vi "Read Components.vi"(8 "error in (no error)":errorcluster, 11 "Snake in":refnum<class "Snake.lvclass">) -> (0 "error out":errorcluster, 2 "Components":T1[](array[typedef]), 3 "Snake out":refnum<class "Snake.lvclass">)   [LabVIEW 2019, in "Snake.lvclass"]
uses:
  Snake.lvclass
  Direction STYP.ctl
  Coordinate STYP.ctl
  private/Snake Component STYP.ctl
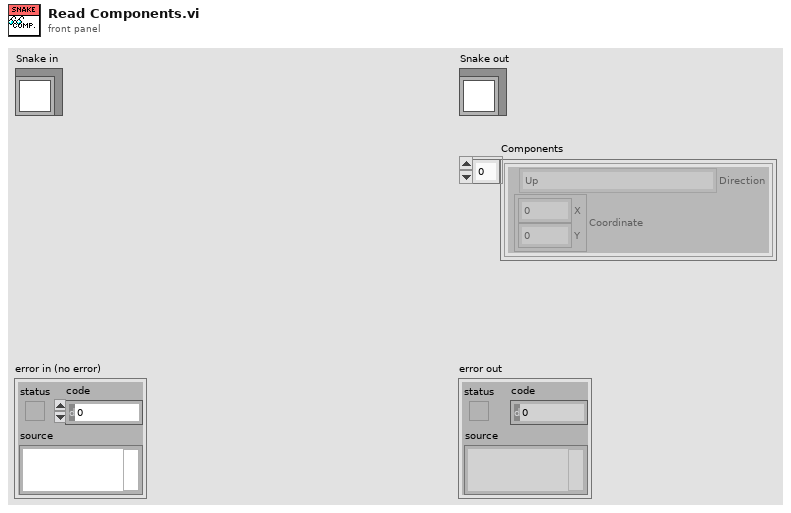
[diagram p1: front panel]
types:
  T1 = typedef "Snake.lvclass/Snake Component STYP.ctl" = cluster{"Direction":T2, "Coordinate":T3}
  T2 = typedef "Direction STYP.ctl" = enum16{"Up", "Down", "Left", "Right"}
  T3 = typedef "Coordinate STYP.ctl" = cluster{"X":i32, "Y":i32}
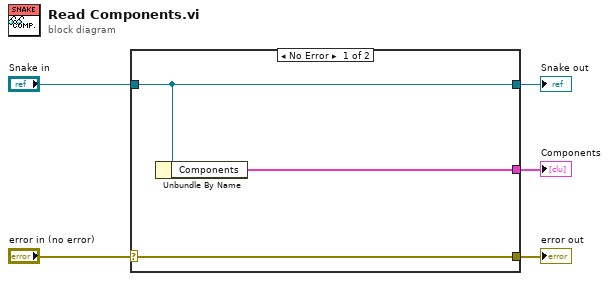
[diagram p0: block diagram]
diagram:
  n1 = case shown="No Error" "error in (no error)" {
    selector: "error in (no error)" -> [w8 w9]
    tunnel: [w8 w9] -> w4
    tunnel: [w7 w10] -> w2
    tunnel: "Snake in" -> [w7 w10]
    tunnel: [w6 _] -> w1
    frame No Error {
      n2 = Unbundle By Name(w7) -> ("Components"=w6:T1[])
    }
    frame Error {
    }
  }
  "error out" <- w4
  "Snake out" <- w2
  "Components" <- w1
